vi "Create Main Message Queues.vi"(8 "error in (no error)":errorcluster, 11 "Process Name":string="Feed Module 1") -> (0 "error out":errorcluster, 3 "Message Queues out":T1)   [LabVIEW 2018]
doc: "This VI creates and initializes all the message queues for your application. If your application requires more than one message queue, right-click the \"Message Queues\" constant above and select Open Type Def. Add the new Message Queue(s) to the type definition, then initialize them in this VI."
uses:
  Main Queue Cluster.ctl
  support/Message Queue/Message Cluster.ctl
  support/Message Queue/Enqueue Message (Single).vi
  support/Message Queue/Message Queue.lvlib
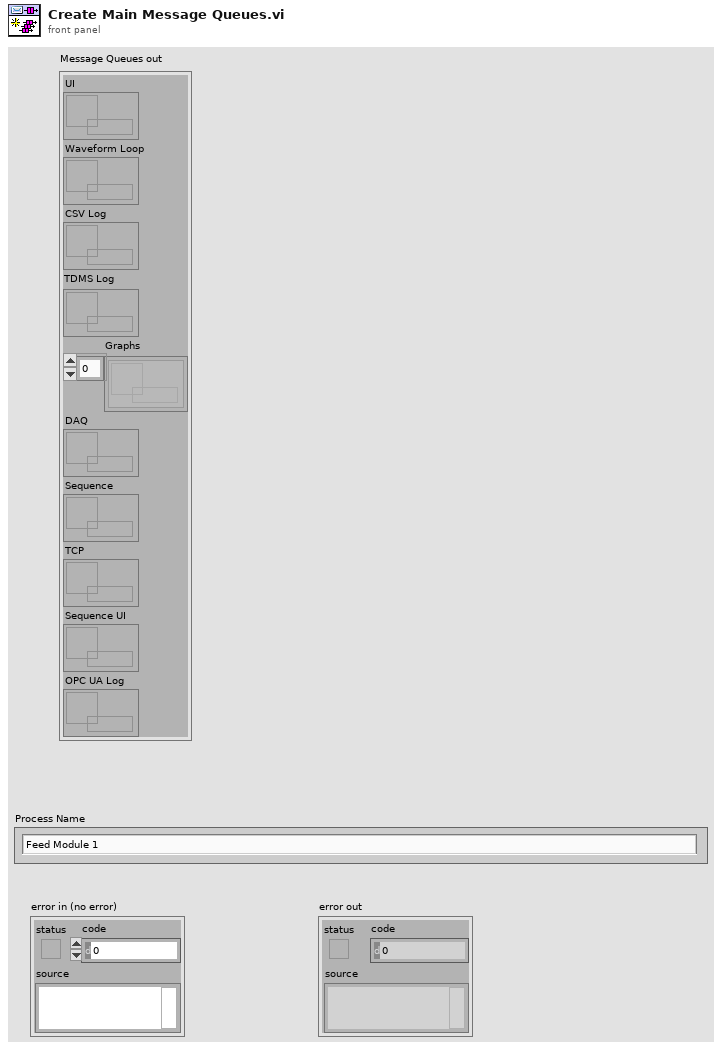
[diagram p1: front panel]
types:
  T1 = typedef "Main Queue Cluster.ctl" = cluster{"UI":refnum<queue>, "Waveform Loop":refnum<queue>, "CSV Log":refnum<queue>, "TDMS Log":refnum<queue>, "Graphs":refnum<queue>[], "DAQ":refnum<queue>, "Sequence":refnum<queue>, "TCP":refnum<queue>, "Sequence UI":refnum<queue>, "OPC UA Log":refnum<queue>}
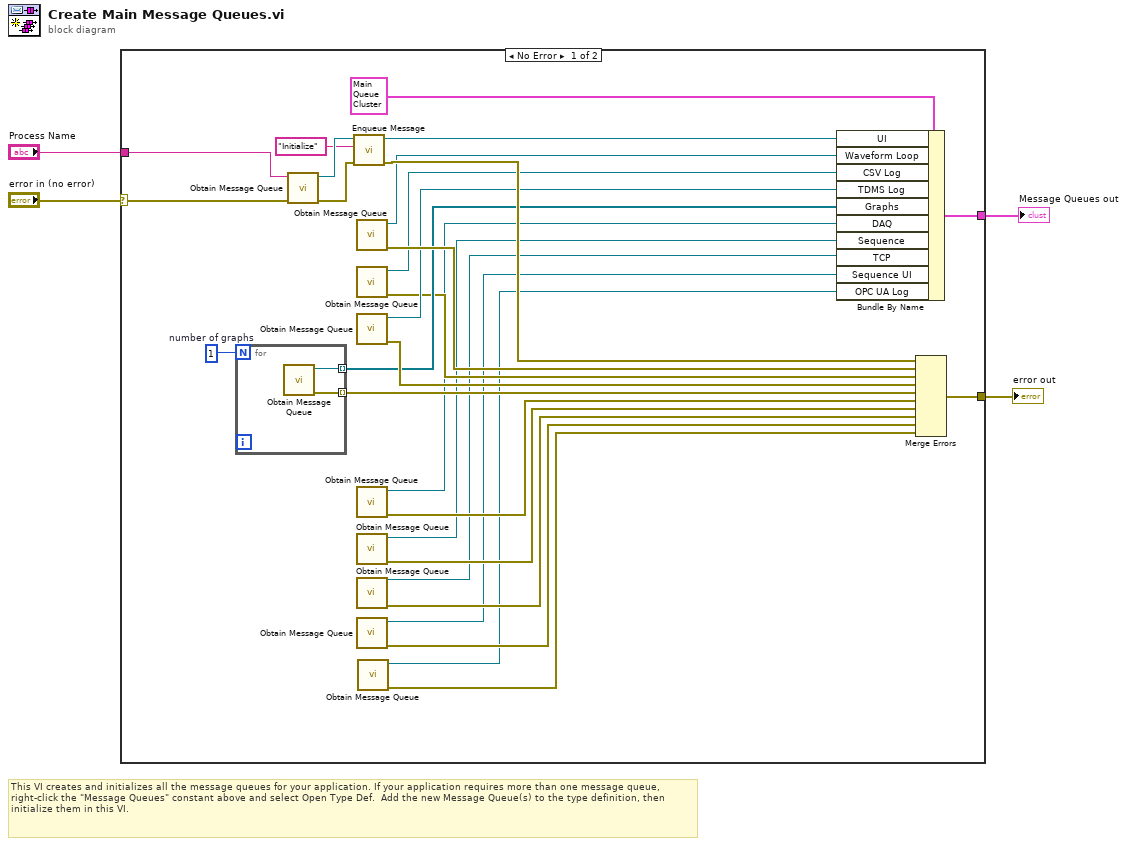
[diagram p0: block diagram]
diagram:
  # "This VI creates and initializes all the message queues for your application. If your application requires more than one message queue, right-click the \"Message Queues\" constant above and select Open Type Def.  Add the new Message Queue(s) to the type definition, then initialize them in this VI."
  n1 = case shown="No Error" "error in (no error)" {
    selector: "error in (no error)" -> [w27 w36]
    tunnel: [w28 w36] -> w4
    tunnel: [w32 _] -> w3
    tunnel: "Process Name" -> [w26 _]
    frame No Error {
      w19 = 1  # number of graphs
      n2 = for {
        N: w19 -> [_]
        tunnel: [w35] -> w18 mode=indexing
        tunnel: [w34] -> w17 mode=indexing
        n3 = call "Obtain Message Queue.vi"() -> ("error out"=w34:errorcluster, "Message Queue"=w35:refnum<queue>)  [unwired: 10 in]
      }
      n4 = call "Obtain Message Queue.vi"("error in (no error)"=w27, "name (unnamed)"=w26) -> ("error out"=w31:errorcluster, "Message Queue"=w30:refnum<queue>)  [unwired: 8 in]
      n5 = call-poly "Enqueue Message.vi"("error in (no error)"=w31, "Message"="Initialize", "Message Queue"=w30) -> ("error out"=w33:errorcluster, "dup Message Queue"=w29:refnum<queue>)  [unwired: 7 in]
      n6 = call "Obtain Message Queue.vi"() -> ("error out"=w22:errorcluster, "Message Queue"=w23:refnum<queue>)  [unwired: 10 in]
      n7 = call "Obtain Message Queue.vi"() -> ("error out"=w15:errorcluster, "Message Queue"=w16:refnum<queue>)  [unwired: 10 in]
      n8 = call "Obtain Message Queue.vi"() -> ("error out"=w21:errorcluster, "Message Queue"=w20:refnum<queue>)  [unwired: 10 in]
      n9 = call "Obtain Message Queue.vi"() -> ("error out"=w13:errorcluster, "Message Queue"=w14:refnum<queue>)  [unwired: 10 in]
      n10 = call "Obtain Message Queue.vi"() -> ("error out"=w11:errorcluster, "Message Queue"=w12:refnum<queue>)  [unwired: 10 in]
      n11 = call "Obtain Message Queue.vi"() -> ("error out"=w9:errorcluster, "Message Queue"=w10:refnum<queue>)  [unwired: 10 in]
      n12 = call "Obtain Message Queue.vi"() -> ("error out"=w7:errorcluster, "Message Queue"=w8:refnum<queue>)  [unwired: 10 in]
      n13 = call "Obtain Message Queue.vi"() -> ("error out"=w5:errorcluster, "Message Queue"=w6:refnum<queue>)  [unwired: 10 in]
      n14 = Bundle By Name(cluster=T1 {"UI"=refnum, "Waveform Loop"=refnum, "CSV Log"=refnum, "TDMS Log"=refnum, "Graphs"=[], "DAQ"=refnum, "Sequence"=refnum, "TCP"=refnum, "Sequence UI"=refnum, "OPC UA Log"=refnum} ("Message Queues out"), "UI"=w29, "Waveform Loop"=w23, "CSV Log"=w16, "TDMS Log"=w20, "Graphs"=w18, "DAQ"=w14, "Sequence"=w12, "TCP"=w10, "Sequence UI"=w8, "OPC UA Log"=w6) -> (w32:T1)
      n15 = Merge Errors(w33, w22, w15, w21, w17, w13, w11, w9, w7, w5) -> (w28:errorcluster)
    }
    frame Error {
    }
  }
  "Message Queues out" <- w3
  "error out" <- w4
